vi "Frontend FPP_Kee_modified.vi"() -> ()   [LabVIEW 2016]
panel:
  in  "Gate 2":T1={"Gate Start"=0.0, "Gate Stop"=2.0, "Gate Step (linear only)"=1.0, "Gate Compliance"=0.0001, "Gate PComp"=0.0, "Range mode"=0, "Range"=6} {"Range" max=11 scale=0.0..11.0; "Range mode" items=["Auto", "Limited", "Fixed"]; "Gate PComp" format="%^.2e"; "Gate Compliance" format="%^.2e"; "Gate Step (linear only)" format="%^.4e"; "Gate Stop" format="%^.4e"; "Gate Start" format="%^.4e"}
  in  "Drain":T2={"Drain Start"=0.0, "Drain Stop"=2.0, "Drain Compliance"=0.0001, "Drain Step"=1.0, "Drain PComp"=0.0, "Range mode"=0, "Range"=6} {"Range" max=11 scale=0.0..11.0; "Range mode" items=["Auto", "Limited", "Fixed"]; "Drain PComp" format="%^.2e"; "Drain Step" format="%^.4e"; "Drain Compliance" format="%^.2e"; "Drain Stop" format="%^.4e"; "Drain Start" format="%^.4e"}
  in  "Gate":T3={"Gate Start"=0.0, "Gate Stop"=2.0, "Gate Step"=1.0, "Gate Compliance"=0.0001, "Gate PComp"=0.0, "Range mode"=0, "Range"=6} {"Range" max=11 scale=0.0..11.0; "Range mode" items=["Auto", "Limited", "Fixed"]; "Gate PComp" format="%^.2e"; "Gate Compliance" format="%^.2e"; "Gate Step" format="%^.4e"; "Gate Stop" format="%^.4e"; "Gate Start" format="%^.4e"}
  in  "Drain 2":T4={"Drain Start"=0.0, "Drain Stop"=2.0, "Drain Compliance"=0.0001, "Drain Step (linear only)"=1.0, "Drain PComp"=0.0, "Range mode"=0, "Range"=6} {"Range" max=11 scale=0.0..11.0; "Range mode" items=["Auto", "Limited", "Fixed"]; "Drain PComp" format="%^.2e"; "Drain Step (linear only)" format="%^.4e"; "Drain Compliance" format="%^.2e"; "Drain Stop" format="%^.4e"; "Drain Start" format="%^.4e"}
  in  "Timings":T5={"integration time"=0, "Short/Long integration time"=0.00064, "hold time (sec)"=0.0, "delay time (sec)"=0.0, "Step Time (0 disables)"=0.0, "sweep method"=0, "Pulse period"=0.005, "Base voltage"=0.0, "Pulse width"=0.0005} {"Pulse width" min=0.0005 max=0.1 step=0.0001 format="%.4f"; "Base voltage" format="%^.4e"; "Pulse period" min=0.005 max=1.0 step=0.0001 format="%.4f"; "sweep method" items=["Continuous", "Pulsed"]; "Step Time (0 disables)" format="%.2f"; "delay time (sec)" format="%.4f"; "hold time (sec)" format="%.4f"; "Short/Long integration time" format="%^.0e"; "integration time" scale=0.0..2.0}
  in  "Panel controls":T6={"Emergency Stop"=refnum, "OutputGraph Max"=1e-05, "Text/Graph (text=false)"=FALSE} {"OutputGraph Max" format="%.2e"}
  in  "Panel Controls":T7={"Emergency Stop"=refnum, "TransGraph Max"=1e-05, "Text/Graph (text=false)"=FALSE} {"TransGraph Max" format="%.2e"}
  in  "Tab Control":enum32{"Characteristics", "Other parameters"}(tab)
  out "XY Graph 2":cluster{"Y data in":dbl[], "X data in":dbl[]}[](graph)
  in  "Integration time (long)":dbl=0.32 min=0.04 max=2.0 step=0.02 format="%.2f"
  in  "Integration time (short)":dbl=0.00064 min=8e-05 max=0.00192 step=8e-05 format="%^.0e"
  in  "Drain Range":u8(slide)=6 max=11 scale=0.0..11.0
  in  "Drain Range mode":u16(ring) items=["Auto", "Limited", "Fixed"]
  in  "Gate Range":u8(slide)=6 max=11 scale=0.0..11.0
  in  "Gate Range mode":u16(ring) items=["Auto", "Limited", "Fixed"]
  in  "Sampling mode":u32(slide) scale=0.0..4.0
  in  "Number of Samples":i32=500 min=0 step=1
  in  "Time":dbl=240.0 min=0.0 format="%.2f"
  in  "Drain":dbl=-10.0 min=-100.0 max=100.0 format="%.2f"
  in  "Gate":dbl=-60.0 min=-100.0 max=100.0 format="%.2f"
  in  "sweep method":u16(ring) items=["Continuous", "Pulsed"]
  out "Id":dbl format="%.2e"
  out "Ig":dbl format="%.2e"
  in  "Sweep Start":bool caption="Sweep start"
  in  "Interrupt run":bool
  in  "Running":bool
  out "Path":path
  in  "integration time":u32(slide)=1 max=2 step=1 scale=0.0..2.0
  in  "sweep mode":u16(ring)=1 items=["Single", "Double"]
  in  "Transfer Start":bool
  in  "Output Start":bool
  in  "Drain: Step":dbl=-1.0 min=-100.0 max=100.0 format="%.2f"
  in  "Drain: Stop":dbl=-60.0 min=-100.0 max=100.0 format="%.2f"
  in  "Drain:Start":dbl min=-100.0 max=100.0 format="%.2f"
  in  "Gate: Step":dbl=-20.0 min=-100.0 max=100.0 format="%.2f"
  in  "Gate: Stop":dbl=-60.0 min=-100.0 max=100.0 format="%.2f"
  in  "Gate: Start":dbl min=-100.0 max=100.0 format="%.2f"
  out "XY Graph":cluster{"Y data in":dbl[], "X data in":dbl[]}[](graph)
  in  "Drain: Compliance":dbl=0.001 min=1e-12 max=0.02 format="%.8f"
  in  "Gate: Compliance":dbl=0.001 min=1e-12 max=0.02 format="%.8f"
  in  "Drain: Step":dbl=-5.0 min=-100.0 max=100.0 format="%.2f"
  in  "Drain: Stop":dbl=-10.0 min=-100.0 max=100.0 format="%.2f"
  in  "Drain:Start":dbl=-5.0 min=-100.0 max=100.0 format="%.2f"
  in  "Gate: Step":dbl=-1.0 min=-100.0 max=100.0 format="%.2f"
  in  "Gate: Stop":dbl=-60.0 min=-100.0 max=100.0 format="%.2f"
  in  "Gate: Start":dbl=10.0 min=-100.0 max=100.0 format="%.2f"
  out "Vp_2":dbl format="%.2e"
  out "Vp_1":dbl format="%.2e"
  out "Delta V":dbl format="%.2e"
  in  "Thickness":dbl=0.00064 min=8e-05 max=100.0 step=1e-07 format="%^.0e"
  out "Conductivity":dbl format="%.2e"
  in  "Pulse width":dbl=0.0005 min=0.0005 max=0.1 step=0.0001 format="%.4f"
  in  "Base voltage":dbl min=-100.0 max=100.0 format="%.2f"
  in  "Pulse period":dbl=0.005 min=0.005 max=1.0 step=0.0001 format="%.4f"
  in  "Drain Power Compliance":dbl min=0.0 max=1.0 format="%.2f"
  in  "Gate Power\nCompliance":dbl min=0.0 max=1.0 format="%.2f"
  in  "OutputGraph Max":dbl=1e-05 format="%.2e"
  in  "TransGraph Max":dbl=1e-05 format="%.2e"
  in  "SPA Display":bool
  in  "Step delay /s":dbl min=0.0 max=1.0 format="%.2f"
  in  "hold time /s":dbl min=0.0 max=655.35 step=0.01 format="%.2f"
  in  "delay time /s":dbl min=0.0 max=65.535 step=0.0001 format="%.2f"
  in  "Decimal places in header":i8=1
  out "error out":errorcluster
  # "Transfer Characteristics"
  # "Stress Measurements"
  # "V"
  # "V"
  # "V"
  # "Gate"
  # "V"
  # "V"
  # "V"
  # "V"
  # "Drain"
  # "V"
  # "Output Characteristics"
  # "s"
  # "V"
  # "V"
  # "V"
  # "Gate"
  # "V"
  # "V"
  # "Drain"
  # "V"
  # "For Four Point Probe measurements ONLY!"
  # "SMU1 = Probe 1\nSMU2 = Drain\nSMU3 = Gate\nSMU4 = Probe 2\nVSU1 = Source"
  # "A"
  # "A"
  # "Vp1"
  # "Vp2"
  # "s"
  # "Pulsed mode settings"
  # "s"
  # "NOTE - THIS OVERRIDES THE COMPLIANCE VALUES!"
  # "A"
  # "A"
  # "Enter max power in Watts (max 1W)"
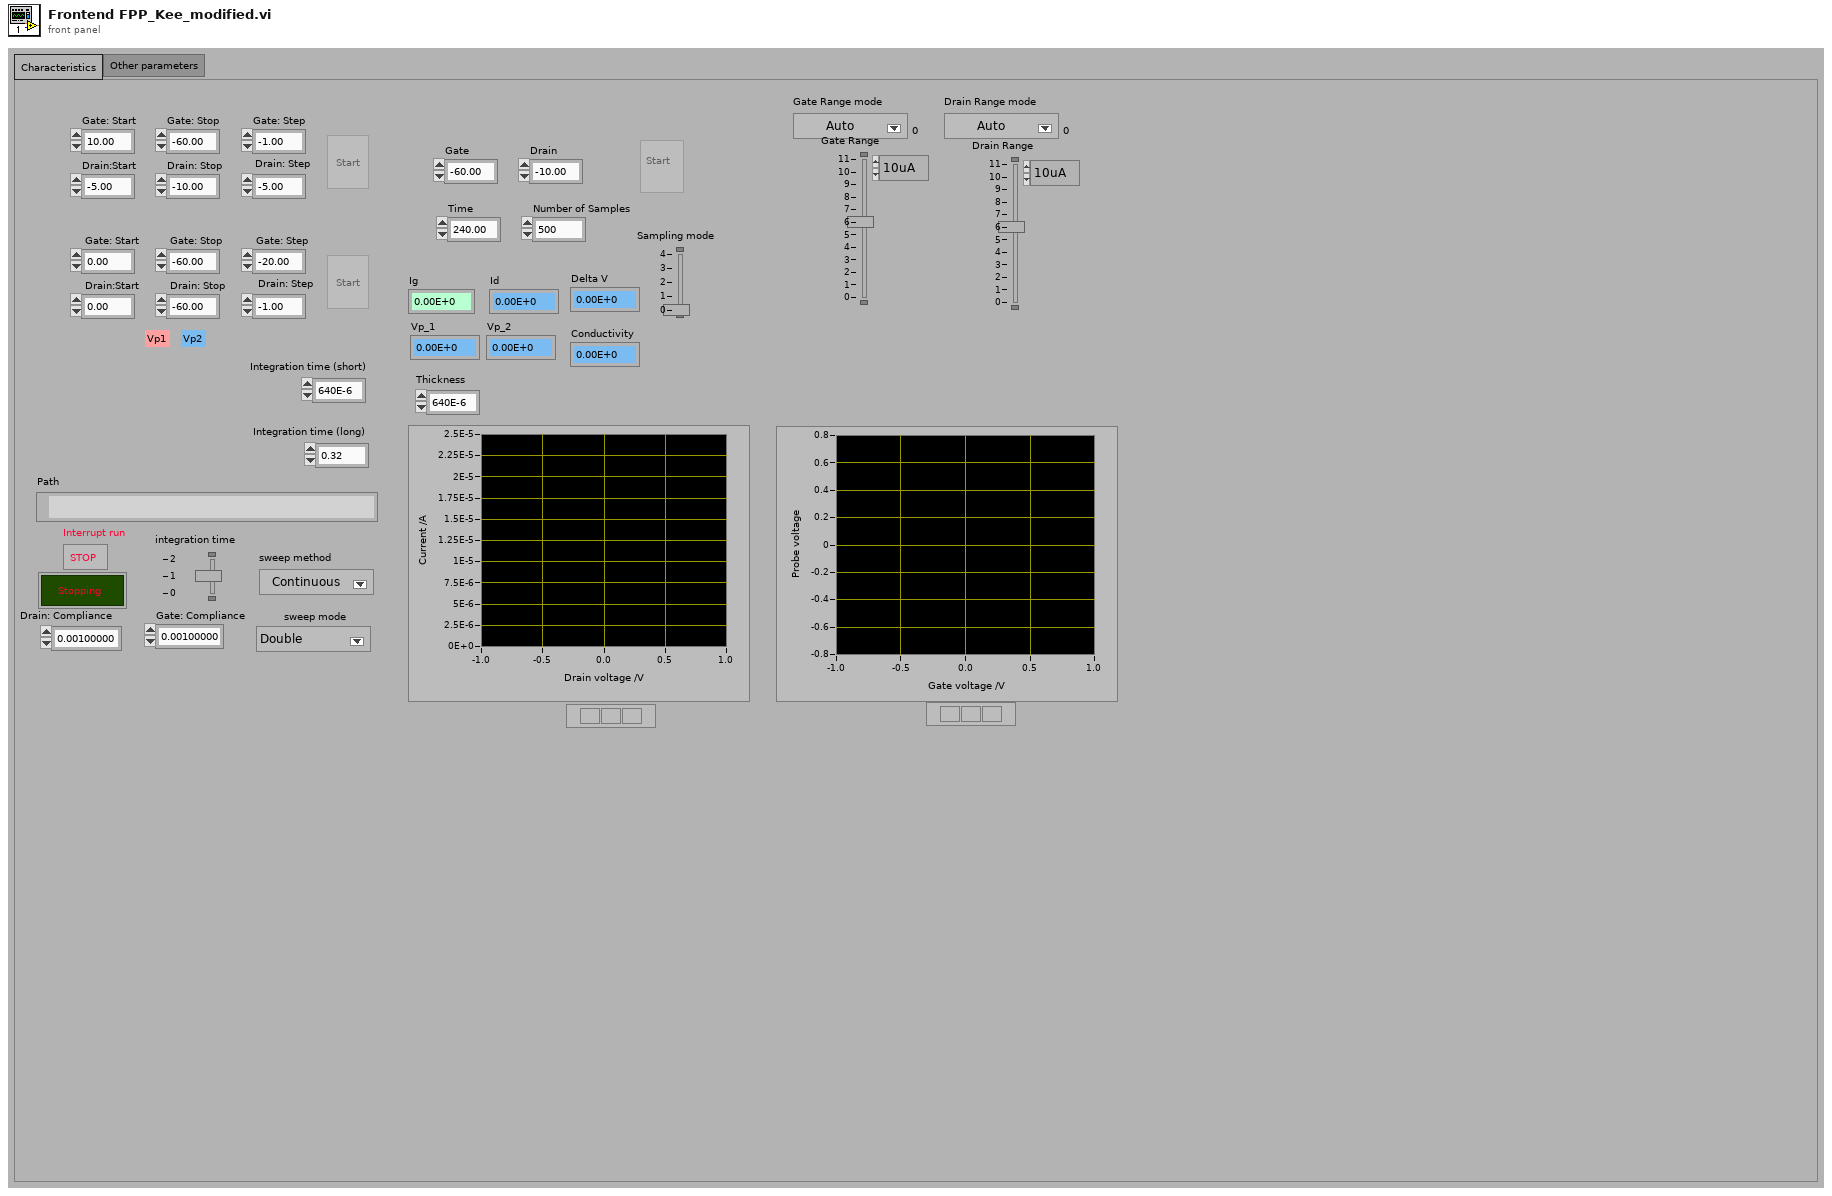
[diagram p1: front panel]
types:
  T1 = cluster{"Gate Start":dbl, "Gate Stop":dbl, "Gate Step (linear only)":dbl, "Gate Compliance":dbl, "Gate PComp":dbl, "Range mode":u16, "Range":u8}
  T2 = cluster{"Drain Start":dbl, "Drain Stop":dbl, "Drain Compliance":dbl, "Drain Step":dbl, "Drain PComp":dbl, "Range mode":u16, "Range":u8}
  T3 = cluster{"Gate Start":dbl, "Gate Stop":dbl, "Gate Step":dbl, "Gate Compliance":dbl, "Gate PComp":dbl, "Range mode":u16, "Range":u8}
  T4 = cluster{"Drain Start":dbl, "Drain Stop":dbl, "Drain Compliance":dbl, "Drain Step (linear only)":dbl, "Drain PComp":dbl, "Range mode":u16, "Range":u8}
  T5 = cluster{"integration time":u32, "Short/Long integration time":dbl, "hold time (sec)":dbl, "delay time (sec)":dbl, "Step Time (0 disables)":dbl, "sweep method":u16, "Pulse period":dbl, "Base voltage":dbl, "Pulse width":dbl}
  T6 = cluster{"Emergency Stop":refnum<vi>, "OutputGraph Max":dbl, "Text/Graph (text=false)":bool}
  T7 = cluster{"Emergency Stop":refnum<vi>, "TransGraph Max":dbl, "Text/Graph (text=false)":bool}
  T8 = cluster{"V2 Start":dbl, "V2 Step":dbl, "Number of points":i32}
  T9 = enum16{"open", "replace", "create", "open or create", "replace or create", "replace or create with confirmation"}
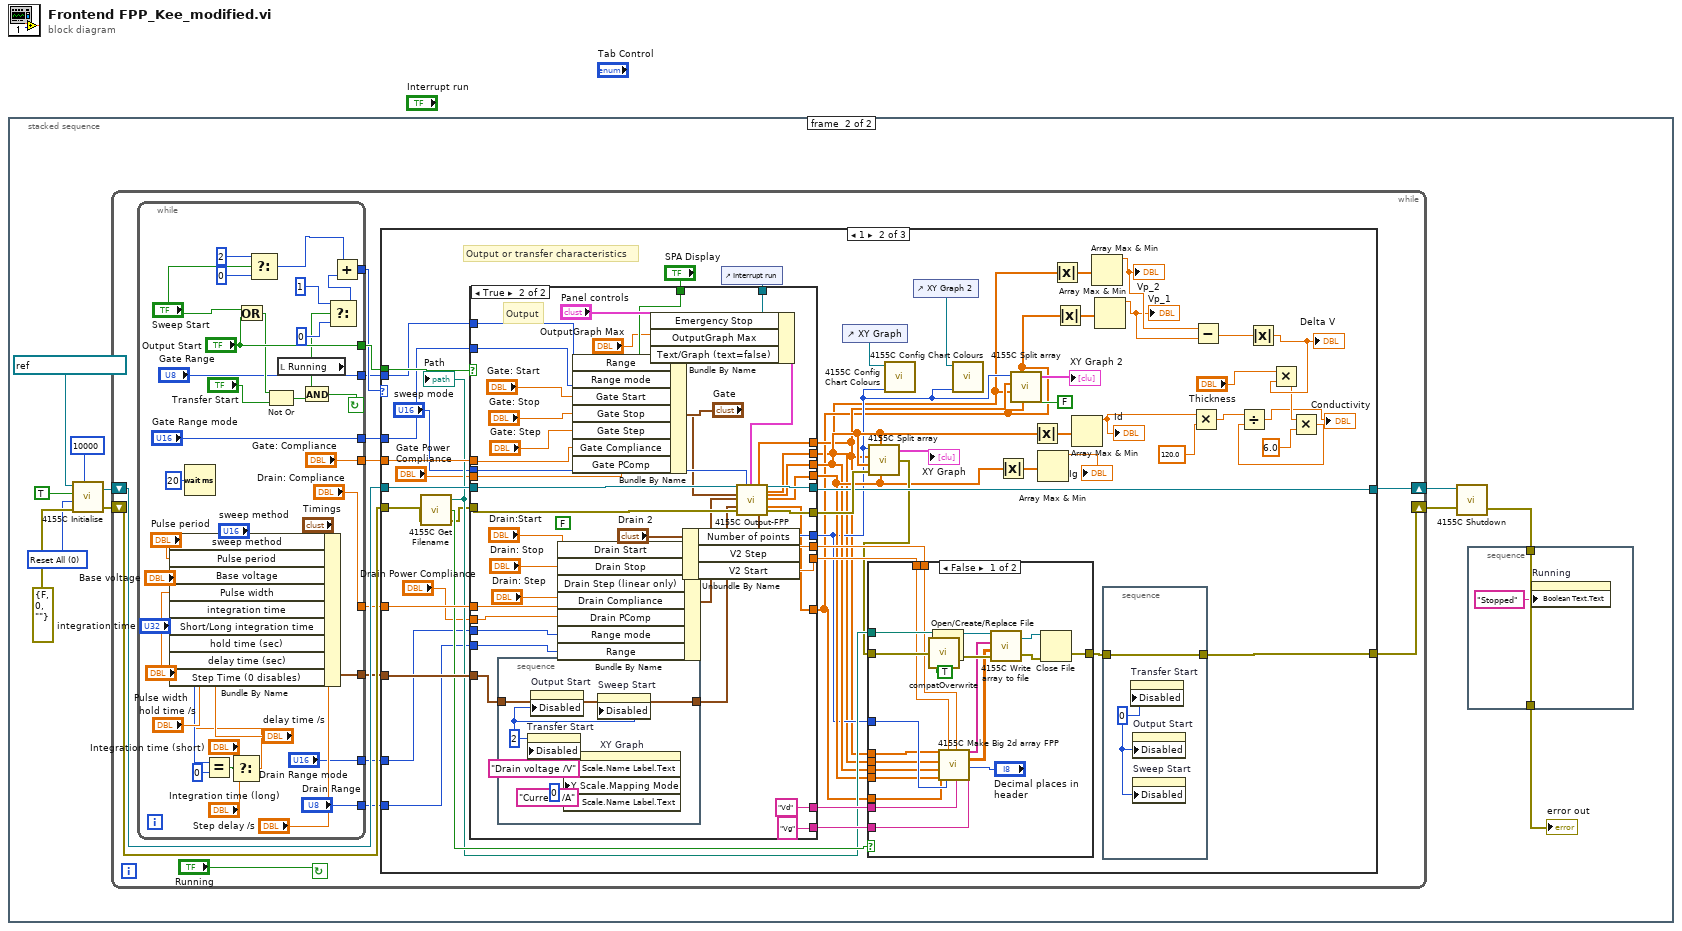
[diagram p0: block diagram]
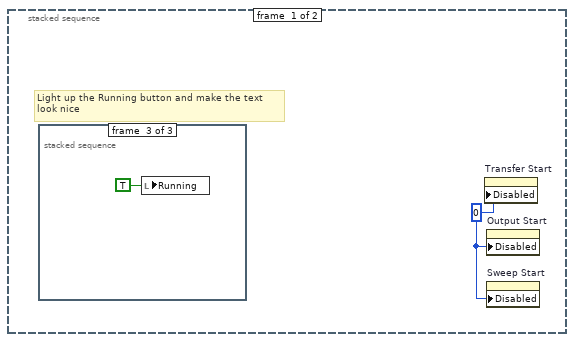
[diagram p2: hidden frame]
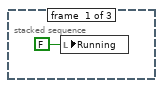
[diagram p3: hidden frame]
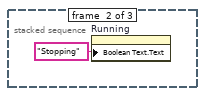
[diagram p4: hidden frame]
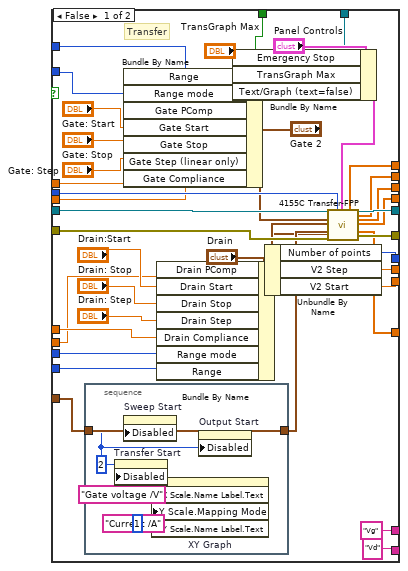
[diagram p7: hidden frame]
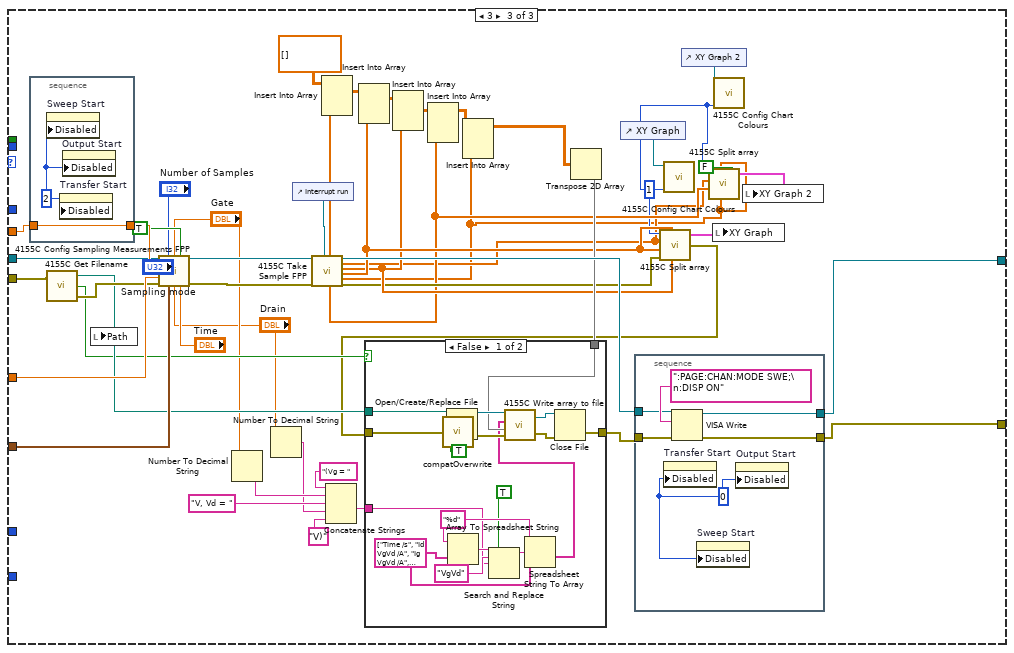
[diagram p8: hidden frame]
diagram:
  n1 = stacked-sequence {
    frame #0 {
      w1 = u8 0 ("Disabled")
      # "Light up the Running button and make the text\nlook nice"
      n2 = stacked-sequence {
        frame #0 {
          n3 = local write "Running"(FALSE ("Running")) -> ()
        }
        frame #1 {
          n4 = property on="Running" class="Bool (strict)"("Boolean Text.Text"="Stopping") -> ()  [unwired: 2 in, 2 out]
        }
        frame #2 {
          (unwired) FALSE ("Running")
          n5 = local write "Running"(TRUE ("Running")) -> ()
        }
      }
      n6 = property on="Transfer Start" class="Bool (strict)"("Disabled"=w1) -> ()  [unwired: 2 in, 2 out]
      n7 = property on="Output Start" class="Bool (strict)"("Disabled"=w1) -> ()  [unwired: 2 in, 2 out]
      n8 = property on="Sweep Start" class="Bool (strict)"("Disabled"=w1) -> ()  [unwired: 2 in, 2 out]
    }
    frame #1 {
      w11 = u16 0 items=["Reset All", "Partial reset"] ("Type of reset")
      n9 = call "4155C Initialise.vi"("VISA resource name in"=refnum<visa-resource-name> "GPIB0::14::INSTR", "Reset"=TRUE, "Type of reset"=w11, "error in (no error)"=errorcluster {"status"=FALSE, "code"=0, "source"=""}, "VISA Timeout Value"=u32 10000) -> ("VISA Resource Name out"=w10:refnum<visa-resource-name>, "error out"=w9:errorcluster)
      n10 = while {
        shift-left: w10 -> [w24]
        shift-right: [w26] -> w5
        shift-left: w9 -> [w25]
        shift-right: [w27] -> w6
        stop <- "Running" continue-if-true
        n11 = while {
          tunnel: ["Gate Range"] -> w16
          tunnel: ["Gate Range mode"] -> w17
          tunnel: ["Drain Range"] -> w18
          tunnel: ["Drain Range mode"] -> w19
          tunnel: ["Drain: Compliance"] -> w20
          tunnel: [w49] -> w21
          tunnel: ["Gate: Compliance"] -> w22
          tunnel: [w55] -> w23
          tunnel: ["Output Start"] -> w28
          stop <- w64 continue-if-true
          n12 = Wait (ms)(milliseconds to wait=u32 20) -> ()  [unwired: 1 out]
          n13 = Equal?(x="integration time", y=u32 0) -> (x = y?=w46:bool)
          n14 = Select(t="Integration time (short)", s=w46, f="Integration time (long)") -> (s? t:f=w43:dbl)
          n15 = Bundle By Name(cluster="Timings", "sweep method"="sweep method", "Pulse period"="Pulse period", "Base voltage"="Base voltage", "Pulse width"="Pulse width", "integration time"="integration time", "Short/Long integration time"=w43, "hold time (sec)"="hold time /s", "delay time (sec)"="delay time /s", "Step Time (0 disables)"="Step delay /s") -> (w49:T5)
          n16 = Or(x="Sweep Start", y="Output Start") -> (x .or. y?=w61:bool)
          n17 = Select(t=i8 2, s="Sweep Start", f=i8 0) -> (s? t:f=w31:i8)
          n18 = Not Or(1:"Transfer Start", 2:w61) -> (0:w63:bool)
          n19 = local read "Running"() -> (w58:bool)
          n20 = And(x=w58, y=w63) -> (x .and. y?=w64:bool)
          n21 = Select(t=i8 1, s=w58, f=i8 0) -> (s? t:f=w54:i8)
          n22 = Add(x=w31, y=w54) -> (x+y=w55:i8)
        }
        n23 = case shown="1" w23 {
          tunnel: w28 -> [_ w122 _]
          tunnel: w21 -> [_ w121 w279]
          tunnel: w22 -> [_ w120 w287]
          tunnel: w20 -> [_ w119 w283]
          tunnel: [w67 w110 w285] -> w27
          tunnel: [w66 w113 w286] -> w26
          tunnel: w25 -> [w67 w104 w274]
          tunnel: w24 -> [w66 w112 w273]
          tunnel: w19 -> [_ w94 _]
          tunnel: w18 -> [_ w93 _]
          tunnel: w17 -> [_ w92 _]
          tunnel: w16 -> [_ w91 _]
          frame 0, Default {
            # "Someone's deselected the running button so just shutdown..."
          }
          frame 1 {
            # "Output or transfer characteristics"
            n24 = call "4155C Get Filename.vi"("error in (no error)"=w104) -> ("error out"=w103:errorcluster, "cancelled"=w109:bool, "path"=w108:path)  [unwired: 2 in]
            "Path" <- w108
            n25 = control-ref of="Interrupt run"() -> (w105:refnum<vi>)
            n26 = case shown="True" w122 {
              tunnel: w112 -> [w174 w220]
              tunnel: w103 -> [w173 w219]
              tunnel: w121 -> [w177 w225]
              tunnel: w120 -> [w183 w232]
              tunnel: w119 -> [w188 w231]
              tunnel: "sweep mode" -> [w182 w230]
              tunnel: [w150 w198] -> w85
              tunnel: [w149 w197] -> w80
              tunnel: [w152 w196] -> w90
              tunnel: [w151 w195] -> w95
              tunnel: [w181 w229] -> w113
              tunnel: [w180 w228] -> w118
              tunnel: [w153 w201] -> w86
              tunnel: [w154 w200] -> w116
              tunnel: [w155 w199] -> w117
              tunnel: ["Vg" "Vd"] -> w115
              tunnel: ["Vd" "Vg"] -> w114
              tunnel: w105 -> [w171 w218]
              tunnel: "SPA Display" -> [w170 w216]
              tunnel: "Drain Power Compliance" -> [w166 w213]
              tunnel: "Gate Power\nCompliance" -> [w167 w212]
              tunnel: w94 -> [w158 w206]
              tunnel: w93 -> [w157 w205]
              tunnel: w92 -> [w159 w204]
              tunnel: w91 -> [w160 w203]
              tunnel: [w148 w194] -> w82
              frame False {
                # "Transfer"
                n27 = stacked-sequence {
                  tunnel: w177 -> [w192]
                  tunnel: [w192] -> w165
                  frame #0 {
                    w190 = u8 2 ("Disabled")
                    n28 = property on="Transfer Start" class="Bool (strict)"("Disabled"=w190) -> ()  [unwired: 2 in, 2 out]
                    n29 = property on="Sweep Start" class="Bool (strict)"("Disabled"=w190) -> ()  [unwired: 2 in, 2 out]
                    n30 = property on="XY Graph" class="XYGraph (strict)"("X Scale.Name Label.Text"="Gate voltage /V", "Y Scale.Mapping Mode"=u8 1, "Y Scale.Name Label.Text"="Current /A") -> ()  [unwired: 2 in, 2 out]
                    n31 = property on="Output Start" class="Bool (strict)"("Disabled"=w190) -> ()  [unwired: 2 in, 2 out]
                  }
                }
                n32 = Bundle By Name(cluster="Gate 2", "Range"=w160, "Range mode"=w159, "Gate PComp"=w167, "Gate Start"="Gate: Start", "Gate Stop"="Gate: Stop", "Gate Step (linear only)"="Gate: Step", "Gate Compliance"=w183) -> (w161:T1)
                n33 = Bundle By Name(cluster="Drain", "Drain PComp"=w166, "Drain Start"="Drain:Start", "Drain Stop"="Drain: Stop", "Drain Step"="Drain: Step", "Drain Compliance"=w188, "Range mode"=w158, "Range"=w157) -> (w163:T2)
                n34 = Bundle By Name(cluster="Panel Controls", "Emergency Stop"=w171, "TransGraph Max"="TransGraph Max", "Text/Graph (text=false)"=w170) -> (w168:T7)
                n35 = call "4155C Transfer-FPP.vi"("VISA resource name in"=w174, "Gate"=w161, "Drain"=w163, "Timings"=w165, "error in (no error)"=w173, "sweep mode"=w182, "Panel Controls"=w168) -> ("VG"=w150:dbl[], "Outparams"=w156:T8, "VISA Resource Name out"=w181:refnum<visa-resource-name>, "Vprobe2"=w149:dbl[], "ID"=w152:dbl[], "IG"=w151:dbl[], "Vprobe1"=w148:dbl[], "error out"=w180:errorcluster)  [unwired: 13 in]
                n36 = Unbundle By Name(w156) -> ("Number of points"=w153:i32, "V2 Step"=w154:dbl, "V2 Start"=w155:dbl)
              }
              frame True {
                (unwired) FALSE ("Logarithmic")
                # "Output"
                n37 = stacked-sequence {
                  tunnel: w225 -> [w238]
                  tunnel: [w238] -> w211
                  frame #0 {
                    w236 = u8 2 ("Disabled")
                    n38 = property on="Transfer Start" class="Bool (strict)"("Disabled"=w236) -> ()  [unwired: 2 in, 2 out]
                    n39 = property on="Output Start" class="Bool (strict)"("Disabled"=w236) -> ()  [unwired: 2 in, 2 out]
                    n40 = property on="XY Graph" class="XYGraph (strict)"("X Scale.Name Label.Text"="Drain voltage /V", "Y Scale.Mapping Mode"=u8 0, "Y Scale.Name Label.Text"="Current /A") -> ()  [unwired: 2 in, 2 out]
                    n41 = property on="Sweep Start" class="Bool (strict)"("Disabled"=w236) -> ()  [unwired: 2 in, 2 out]
                  }
                }
                n42 = Bundle By Name(cluster="Drain 2", "Drain Start"="Drain:Start", "Drain Stop"="Drain: Stop", "Drain Step (linear only)"="Drain: Step", "Drain Compliance"=w231, "Drain PComp"=w213, "Range mode"=w206, "Range"=w205) -> (w209:T4)
                n43 = Bundle By Name(cluster="Gate", "Range"=w203, "Range mode"=w204, "Gate Start"="Gate: Start", "Gate Stop"="Gate: Stop", "Gate Step"="Gate: Step", "Gate Compliance"=w232, "Gate PComp"=w212) -> (w207:T3)
                n44 = Bundle By Name(cluster="Panel controls", "Emergency Stop"=w218, "OutputGraph Max"="OutputGraph Max", "Text/Graph (text=false)"=w216) -> (w214:T6)
                n45 = call "4155C Output-FPP.vi"("VISA resource name in"=w220, "Gate"=w207, "Drain"=w209, "Timings"=w211, "error in (no error)"=w219, "sweep mode"=w230, "Panel controls"=w214) -> ("VD"=w198:dbl[], "Outparams"=w202:T8, "VISA Resource Name out"=w229:refnum<visa-resource-name>, "Vprobe2"=w197:dbl[], "ID"=w196:dbl[], "IG"=w195:dbl[], "Vprobe1"=w194:dbl[], "error out"=w228:errorcluster)  [unwired: 13 in]
                n46 = Unbundle By Name(w202) -> ("Number of points"=w201:i32, "V2 Step"=w200:dbl, "V2 Start"=w199:dbl)
              }
            }
            n47 = control-ref of="XY Graph"() -> (w106:refnum<vi>)
            n48 = call "4155C Split array.vi"("Number of VAR2 steps"=w86, "Y2 data in"=w90, "X data in"=w85, "Y1 data in"=w90, "Y3 data in"=w95, "error in (no error)"=w118) -> ("Array of clusters"=→"XY Graph":cluster{"Y data in":dbl[], "X data in":dbl[]}[], "error out"=w102:errorcluster)  [unwired: 1 in]
            n49 = case shown="False" w109 {
              tunnel: w102 -> [w145 w147]
              tunnel: [w140 w147] -> w111
              tunnel: w108 -> [w144 _]
              tunnel: w86 -> [w138 _]
              tunnel: w90 -> [w128 _]
              tunnel: w85 -> [w130 _]
              tunnel: w80 -> [w129 _]
              tunnel: w95 -> [w127 _]
              tunnel: w117 -> [w132 _]
              tunnel: w116 -> [w133 _]
              tunnel: w115 -> [w137 _]
              tunnel: w114 -> [w136 _]
              tunnel: w82 -> [w126 _]
              frame False {
                n50 = call <vilib>:"compatOverwrite.vi"("overwrite (F)"=TRUE) -> ("overwrite?"=w125:T9)
                n51 = Open/Create/Replace File(file path (use dialog)=w144, error in=w145, operation (0:open)=w125) -> (refnum out=w142:refnum<file>, error out=w143:errorcluster)  [unwired: 3 in, 1 out]
                n52 = call "4155C Make Big 2d array FPP.vi"("1D Var1"=w130, "1d ID"=w128, "1d Vp2"=w129, "1d IG"=w127, "1d Vp1"=w126, "VAR2 START"=w132, "Number of VAR2 steps"=w138, "VAR2 STEP"=w133, "VAR1 Name"=w137, "Decimal places in header"="Decimal places in header", "VAR2 Name"=w136) -> ("Header array"=w134:string[], "Data array"=w135:dbl[][])  [unwired: 15 in]
                n53 = call "4155C Write array to file.vi"("Byte Stream File Refnum"=w142, "Header"=w134, "Data Array"=w135, "error in (no error)"=w143) -> ("dup refnum"=w139:refnum<file>, "error out"=w141:errorcluster)  [unwired: 1 in]
                n54 = Close File(refnum=w139, error in=w141) -> (error out=w140:errorcluster)  [unwired: 1 out]
              }
              frame True {
              }
            }
            n55 = call "4155C Config Chart Colours.vi"("Numeric"=w86, "XY Graph 2"=w106) -> ()  [unwired: 6 in]
            n56 = control-ref of="XY Graph 2"() -> (w88:refnum<vi>)
            n57 = call "4155C Config Chart Colours.vi"("Numeric"=w86, "XY Graph 2"=w88) -> ()  [unwired: 6 in]
            n58 = Absolute Value(x=w95) -> (abs(x)=w97:dbl[])
            n59 = call "4155C Split array.vi"("Number of VAR2 steps"=w86, "Y2 data in"=w82, "X data in"=w85, "Y1 data in"=w80, "Y3 data in"=w82, "Absolute val?"=FALSE) -> ("Array of clusters"=→"XY Graph 2":cluster{"Y data in":dbl[], "X data in":dbl[]}[])  [unwired: 1 in, 1 out]
            n60 = Absolute Value(x=w90) -> (abs(x)=w96:dbl[])
            n61 = Array Max & Min(array=w97) -> (max value=→"Ig":dbl)  [unwired: 3 out]
            n62 = Absolute Value(x=w80) -> (abs(x)=w81:dbl[])
            n63 = Absolute Value(x=w82) -> (abs(x)=w83:dbl[])
            n64 = Array Max & Min(array=w96) -> (max value=w75:dbl)  [unwired: 3 out]
            "Id" <- w75
            n65 = Array Max & Min(array=w81) -> (max value=w79:dbl)  [unwired: 3 out]
            "Vp_2" <- w79
            n66 = Array Max & Min(array=w83) -> (max value=w78:dbl)  [unwired: 3 out]
            "Vp_1" <- w78
            n67 = stacked-sequence {
              tunnel: w111 -> [w124]
              tunnel: [w124] -> w110
              frame #0 {
                w123 = u8 0 ("Disabled")
                n68 = property on="Transfer Start" class="Bool (strict)"("Disabled"=w123) -> ()  [unwired: 2 in, 2 out]
                n69 = property on="Output Start" class="Bool (strict)"("Disabled"=w123) -> ()  [unwired: 2 in, 2 out]
                n70 = property on="Sweep Start" class="Bool (strict)"("Disabled"=w123) -> ()  [unwired: 2 in, 2 out]
              }
            }
            n71 = Multiply(x=w75, y=120.0) -> (x*y=w74:dbl)
            n72 = Subtract(x=w79, y=w78) -> (x-y=w77:dbl)
            n73 = Absolute Value(x=w77) -> (abs(x)=w72:dbl)
            "Delta V" <- w72
            n74 = Multiply(x="Thickness", y=w72) -> (x*y=w71:dbl)
            n75 = Multiply(x=w71, y=6.0) -> (x*y=w69:dbl)
            n76 = Divide(x=w74, y=w69) -> (x/y=→"Conductivity":dbl)
          }
          frame 3 {
            w243 = 1 ("Numeric")
            n77 = stacked-sequence {
              tunnel: w287 -> [w314]
              tunnel: [w314] -> w284
              frame #0 {
                w313 = u8 2 ("Disabled")
                n78 = property on="Sweep Start" class="Bool (strict)"("Disabled"=w313) -> ()  [unwired: 2 in, 2 out]
                n79 = property on="Transfer Start" class="Bool (strict)"("Disabled"=w313) -> ()  [unwired: 2 in, 2 out]
                n80 = property on="Output Start" class="Bool (strict)"("Disabled"=w313) -> ()  [unwired: 2 in, 2 out]
              }
            }
            n81 = call "4155C Get Filename.vi"("error in (no error)"=w274) -> ("error out"=w272:errorcluster, "cancelled"=w263:bool, "path"=w264:path)  [unwired: 2 in]
            n82 = local write "Path"(w264) -> ()
            n83 = call "4155C Config Sampling Measurements FPP.vi"("VISA session"=w273, "Num Points"="Number of Samples", "Vg"="Gate", "Display on/off"=TRUE, "Gate Compliance"=w284, "Sampling mode"="Sampling mode", "Drain Compliance"=w283, "error in (no error)"=w272, "Timings"=w279, "Vd"="Drain", "Sample time"="Time") -> ("dup VISA resource name"=w280:refnum<visa-resource-name>, "error out"=w281:errorcluster)  [unwired: 3 in]
            n84 = Number To Decimal String(number="Gate") -> (decimal integer string=w261:string)  [unwired: 1 in]
            n85 = Number To Decimal String(number="Drain") -> (decimal integer string=w259:string)  [unwired: 1 in]
            n86 = control-ref of="Interrupt run"() -> (w275:refnum<vi>)
            n87 = call "4155C Take Sample FPP.vi"("VISA resource name in"=w280, "error in (no error)"=w281, "Emergency Stop"=w275) -> ("Time"=w241:dbl[], "Vp1"=w245:dbl[], "VISA Resource Name out"=w282:refnum<visa-resource-name>, "Ig"=w253:dbl[], "Id"=w254:dbl[], "Vp2"=w240:dbl[], "error out"=w252:errorcluster)  [unwired: 10 in]
            n88 = Insert Into Array(array=dbl[][] [] ("Input Array"), new element=w241) -> (w271:dbl[][])  [unwired: 2 in]
            n89 = Concatenate Strings("(Vg = " ("Substring"), w261, "V, Vd = " ("Substring"), w259, "V)" ("Substring")) -> (w257:string)
            n90 = Insert Into Array(array=w271, new element=w254) -> (w270:dbl[][])  [unwired: 2 in]
            n91 = Insert Into Array(array=w270, new element=w253) -> (w269:dbl[][])  [unwired: 2 in]
            n92 = Insert Into Array(array=w269, new element=w245) -> (w267:dbl[][])  [unwired: 2 in]
            n93 = Insert Into Array(array=w267, new element=w240) -> (w247:dbl[][])  [unwired: 2 in]
            n94 = Transpose 2D Array(2D array=w247) -> (transposed array=w265:dbl[][])
            n95 = control-ref of="XY Graph"() -> (w256:refnum<vi>)
            n96 = call "4155C Split array.vi"("Number of VAR2 steps"=w243, "Y2 data in"=w254, "X data in"=w241, "Y1 data in"=w254, "Y3 data in"=w253, "error in (no error)"=w252) -> ("Array of clusters"=w255:cluster{"Y data in":dbl[], "X data in":dbl[]}[], "error out"=w251:errorcluster)  [unwired: 1 in]
            n97 = case shown="False" w263 {
              tunnel: w251 -> [w304 w306]
              tunnel: [w299 w306] -> w266
              tunnel: w264 -> [w303 _]
              tunnel: w265 -> [w297 _]
              tunnel: w257 -> [w289 _]
              frame False {
                w290 = string[] ["Time /s", "Id VgVd /A", "Ig VgVd /A", "Vp1 VgVd /V", "Vp2 VgVd /V"] ("Header")
                w294 = "%d" ("format string")
                n98 = call <vilib>:"compatOverwrite.vi"("overwrite (F)"=TRUE) -> ("overwrite?"=w288:T9)
                n99 = Open/Create/Replace File(file path (use dialog)=w303, error in=w304, operation (0:open)=w288) -> (refnum out=w301:refnum<file>, error out=w302:errorcluster)  [unwired: 3 in, 1 out]
                n100 = Array To Spreadsheet String(array=w290, 3:w294) -> (spreadsheet string=w296:string)  [unwired: 1 in]
                n101 = Search and Replace String(replace all?=TRUE ("replace all? (F)"), input string=w296, search string="VgVd", replace string=w289) -> (result string=w292:string)  [unwired: 4 in, 3 out]
                n102 = Spreadsheet String To Array(format string=w294, spreadsheet string=w292, array type (2D Dbl)=w290) -> (array=w291:string[])  [unwired: 1 in]
                n103 = call "4155C Write array to file.vi"("Byte Stream File Refnum"=w301, "Header"=w291, "Data Array"=w297, "error in (no error)"=w302) -> ("dup refnum"=w298:refnum<file>, "error out"=w300:errorcluster)  [unwired: 1 in]
                n104 = Close File(refnum=w298, error in=w300) -> (error out=w299:errorcluster)  [unwired: 1 out]
              }
              frame True {
              }
            }
            n105 = stacked-sequence {
              tunnel: [w309] -> w286
              tunnel: [w308] -> w285
              tunnel: w282 -> [w311]
              tunnel: w266 -> [w310]
              frame #0 {
                w307 = u8 0 ("Disabled")
                n106 = property on="Transfer Start" class="Bool (strict)"("Disabled"=w307) -> ()  [unwired: 2 in, 2 out]
                n107 = VISA Write(VISA resource name=w311, write buffer=":PAGE:CHAN:MODE SWE;\n:DISP ON" ("write buffer (\"\")"), error in (no error)=w310) -> (VISA resource name out=w309:refnum<visa-resource-name>, error out=w308:errorcluster)  [unwired: 1 out]
                n108 = property on="Sweep Start" class="Bool (strict)"("Disabled"=w307) -> ()  [unwired: 2 in, 2 out]
                n109 = property on="Output Start" class="Bool (strict)"("Disabled"=w307) -> ()  [unwired: 2 in, 2 out]
              }
            }
            n110 = call "4155C Config Chart Colours.vi"("Numeric"=w243, "XY Graph 2"=w256) -> ()  [unwired: 6 in]
            n111 = control-ref of="XY Graph 2"() -> (w246:refnum<vi>)
            n112 = call "4155C Split array.vi"("Number of VAR2 steps"=w243, "Y2 data in"=w240, "X data in"=w241, "Y1 data in"=w245, "Y3 data in"=w240, "Absolute val?"=FALSE) -> ("Array of clusters"=w244:cluster{"Y data in":dbl[], "X data in":dbl[]}[])  [unwired: 1 in, 1 out]
            n113 = local write "XY Graph"(w255) -> ()
            n114 = call "4155C Config Chart Colours.vi"("Numeric"=w243, "XY Graph 2"=w246) -> ()  [unwired: 6 in]
            n115 = local write "XY Graph 2"(w244) -> ()
          }
        }
      }
      n116 = call "4155C Shutdown.vi"("VISA resource name in"=w5, "error in (no error)"=w6) -> ("error out"=w8:errorcluster)  [unwired: 4 in]
      n117 = stacked-sequence {
        tunnel: w8 -> [w316]
        tunnel: [w316] -> w7
        frame #0 {
          n118 = property on="Running" class="Bool (strict)"("Boolean Text.Text"="Stopped") -> ()  [unwired: 2 in, 2 out]
        }
      }
      "error out" <- w7
    }
  }
